vi "XY Graph Set TipStrip String.vi"(8 "error in (no error)":errorcluster, 10 "TipStrip String":string, 11 "XY Graph Refnum":T1) -> (0 "error out":errorcluster, 2 "TipStrip Refnum":refnum<vi>, 3 "XY Graph Refnum (dup)":T1)   [LabVIEW 2021, in "XY Graph Add-Ons.lvlib"]
uses:
  XY Graph Add-Ons.lvlib
  XY Graph Refnum.ctl
  XY Graph Property Tag List.ctl
  7791d90f-93c4-456f-91dc-950c551374c4.vi
  <vilib>/UserTags/UserTags.lvlib
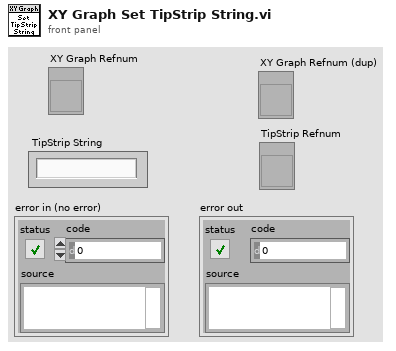
[diagram p1: front panel]
types:
  T1 = typedef "XY Graph Add-Ons.lvlib/XY Graph Refnum.ctl" = refnum<vi>
  T2 = typedef "XY Graph Add-Ons.lvlib/XY Graph Property Tag List.ctl" = enum16{"Max Legend Size", "Preserved Plots", "XScales.GridColors", "YScales.GridColors", "TipStrip String", "TipStrip Visible", "Tool Panels Visibility", "Plots Metadata"}
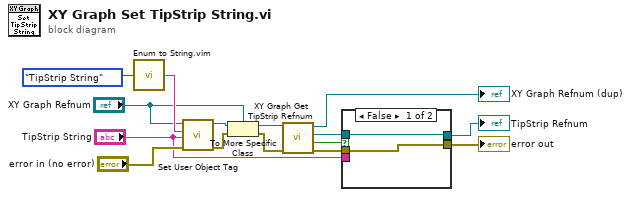
[diagram p0: block diagram]
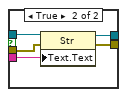
[diagram p2: hidden frame]
diagram:
  n1 = call "Enum to String.vim"("Enum"=XY_Graph_Property_Tag_List."TipStrip String" ("XY Graph Property Tag")) -> ("String"=w14:string)
  n2 = call <vilib>:"Set User Object Tag.vi"("error in (no error)"="error in (no error)", "Value"="TipStrip String", "Tag Name"=w14, "Generic Refnum"="XY Graph Refnum") -> ("error out"=w10:errorcluster, "dup Generic Refnum"=w12:refnum<vi>)  [unwired: 5 in, 1 out]
  n3 = To More Specific Class(target class="XY Graph Refnum", reference=w12, error in=w10) -> (specific class reference=w9:T1, error out=w7:errorcluster)
  n4 = call "XY Graph Get TipStrip Refnum.vi"("Error In"=w7, "XYGraph Refnum"=w9) -> ("Error Out"=w5:errorcluster, "TipStrip Refnum Found?"=w2:bool, "TipStrip Refnum"=w6:refnum<vi>, "XYGraph Refnum"=→"XY Graph Refnum (dup)":T1)  [unwired: 6 in]
  n5 = case shown="False" w2 {
    tunnel: w6 -> [w16 w22]
    tunnel: w5 -> [w17 w21]
    tunnel: "TipStrip String" -> [_ w20]
    tunnel: [w17 w19] -> w3
    tunnel: [w16 w18] -> w1
    frame False {
    }
    frame True {
      n6 = property class="Str"(reference=w22, error in=w21, "Text.Text"=w20) -> (reference out=w18:refnum<vi>, error out=w19:errorcluster)
    }
  }
  "error out" <- w3
  "TipStrip Refnum" <- w1
